vi "open any type of file.vi"(0 "路径 2":path) -> ()   [LabVIEW 2023]
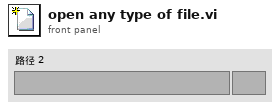
[diagram p1: front panel]
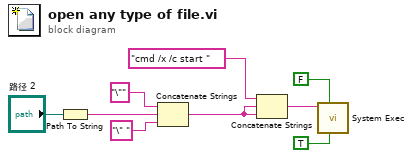
[diagram p0: block diagram]
diagram:
  n1 = Path To String(path="路径 2") -> (string=w8:string)
  n2 = Concatenate Strings("\"" ("字符串"), w8, "\" " ("字符串")) -> (w5:string)
  n3 = Concatenate Strings("cmd /x /c start " ("字符串"), w5, w5) -> (w3:string)
  n4 = call <vilib>:"System Exec.vi"("run minimized? (F)"=TRUE, "wait until completion? (T)"=FALSE, "command line"=w3) -> ()  [unwired: 5 in, 4 out]
